vi "RAW TO DBL.vi"(11 "data in":string) -> (1 "Array":string[](array[string]), 2 "Data regiter (SGL)":sgl[](array[numeric]), 3 "number":dbl[](array[numeric]))   [LabVIEW 2023]
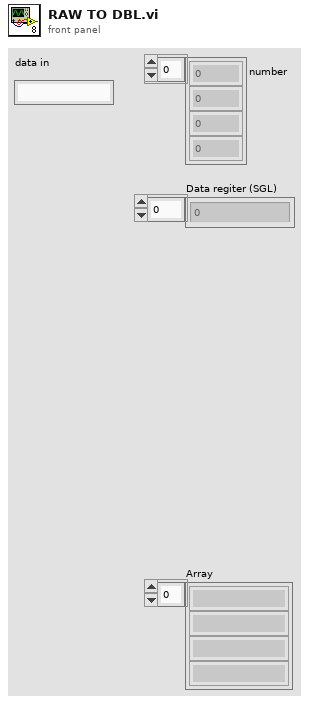
[diagram p1: front panel]
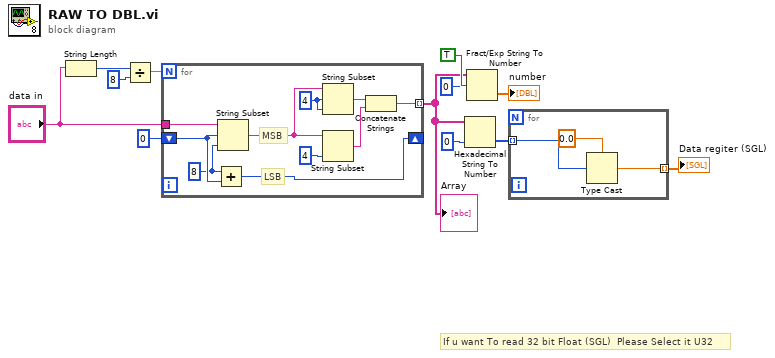
[diagram p0: block diagram]
diagram:
  # "If u want To read 32 bit Float (SGL)  Please Select it U32"
  n1 = String Length(string="data in") -> (length=w5:i32)
  n2 = Divide(x=w5, y=8) -> (x/y=w8:dbl)
  n3 = for {
    N: w8 -> [_]
    tunnel: "data in" -> [w22]
    shift-right: [w21] -> _
    shift-left: 0 ("length (rest)") -> [w20]
    tunnel: [w13] -> w3 mode=indexing
    w17 = 4 ("offset (0)")
    w19 = 8 ("x")
    # "MSB"
    # "LSB"
    n4 = Add(x=w19, y=w20) -> (x+y=w21:i32)
    n5 = String Subset(string=w22, offset (0)=w20, length (rest)=w19) -> (substring=w14:string)
    n6 = String Subset(string=w14, offset (0)=w17, length (rest)=w17) -> (substring=w16:string)
    n7 = String Subset(string=w14, length (rest)=4 ("length (rest)")) -> (substring=w15:string)  [unwired: 1 in]
    n8 = Concatenate Strings(w16, w15) -> (w13:string)
  }
  "Array" <- w3
  n9 = Hexadecimal String To Number(string=w3, default (0uL)=u32 0 ("default (0 U32)")) -> (number=w1:u32[])  [unwired: 1 in, 1 out]
  n10 = Fract/Exp String To Number(use system decimal point (T)=TRUE, string=w3, offset=0) -> (number=→"number":dbl[])  [unwired: 1 in, 1 out]
  n11 = for {
    tunnel: [w24] -> w2 mode=indexing
    tunnel: w1 -> [w23] mode=indexing
    n12 = Type Cast(type=sgl 0.0 ("default (0 U32)"), x=w23) -> (*(type *) &x=w24:sgl)
  }
  "Data regiter (SGL)" <- w2
